vi "Edit.vi"(8 "error in (no error)":errorcluster, 10 "Edit dialog":T1, 11 "Action in":refnum<class "Move-Relative.lvclass">) -> (0 "error out":errorcluster, 3 "Action out":refnum<class "Move-Relative.lvclass">)   [LabVIEW 2013, in "PowderDeposition.lvlib" / "Move-Relative.lvclass"]
uses:
  Move-Relative.lvclass
  Move-Relative-settings.ctl
  Move-Relative.lvclass/Move-Relative.ctl
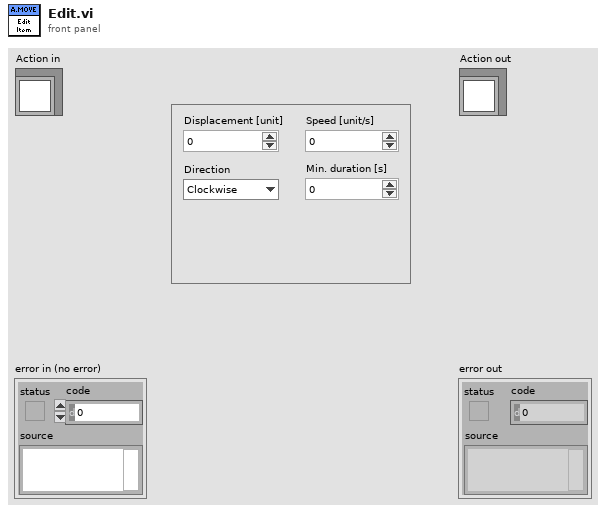
[diagram p1: front panel]
types:
  T1 = typedef "PowderDeposition.lvlib/Move-Relative.lvclass/Move-Relative-settings.ctl" = cluster{"Displacement":dbl, "Speed":dbl, "Direction":enum16{"Clockwise", "Counter-clockwise"}, "Min duration":dbl}
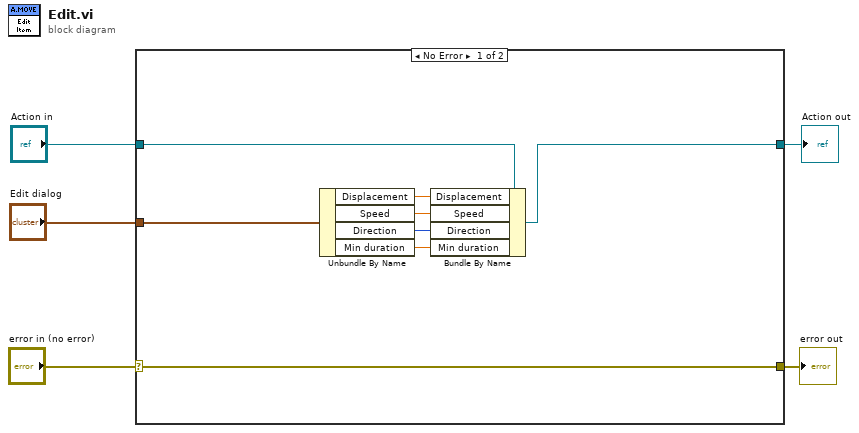
[diagram p0: block diagram]
diagram:
  n1 = case shown="No Error" "error in (no error)" {
    selector: "error in (no error)" -> [w6 w15]
    tunnel: [w6 w15] -> w4
    tunnel: [w7 w14] -> w2
    tunnel: "Action in" -> [w8 w14]
    tunnel: "Edit dialog" -> [w9 _]
    frame No Error {
      n2 = Unbundle By Name(w9) -> ("Displacement"=w13:dbl, "Speed"=w12:dbl, "Direction"=w11:enum16{"Clockwise", "Counter-clockwise"}, "Min duration"=w10:dbl)
      n3 = Bundle By Name(cluster=w8, "Displacement"=w13, "Speed"=w12, "Direction"=w11, "Min duration"=w10) -> (w7:refnum<class "Move-Relative.lvclass">)
    }
    frame Error {
    }
  }
  "error out" <- w4
  "Action out" <- w2
